vi "onHttpDelete.vi"(6 "timeout":i32=10000, 7 "output file":path, 8 "error in":errorcluster, 10 "url":string, 11 "advanced-http-client in":refnum<class "advanced-http-client.lvclass">) -> (0 "error out":errorcluster, 1 "body":string, 2 "headers":string, 3 "advanced-http-client out":refnum<class "advanced-http-client.lvclass">)   [LabVIEW 2020, in "REST Client.lvlib" / "advanced-http-client.lvclass"]
uses:
  advanced-http-client.lvclass
  advanced-http-client.lvclass/advanced-http-client.ctl
  <vilib>/NI/Advanced HTTP Client/Session.lvclass
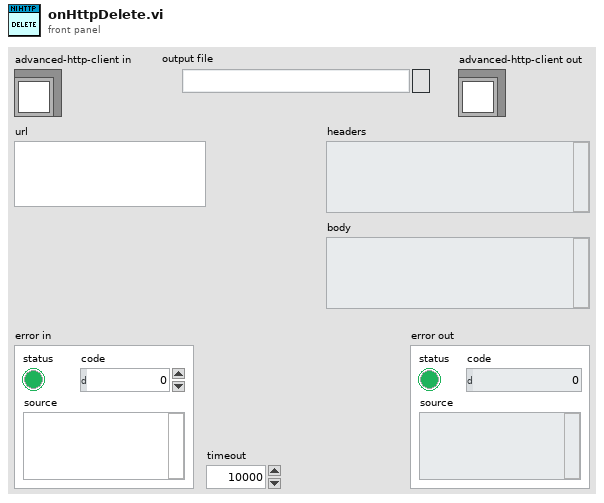
[diagram p1: front panel]
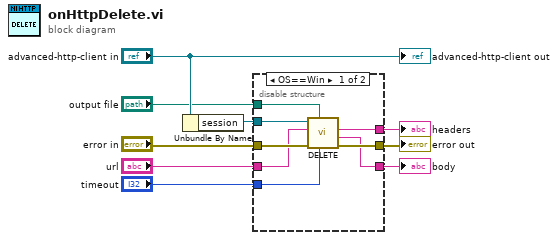
[diagram p0: block diagram]
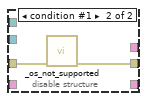
[diagram p2: hidden frame]
diagram:
  n1 = Unbundle By Name("advanced-http-client in") -> ("session"=w8:refnum<class "Session.lvclass">)
  n2 = disable-structure shown="OS==Win" {
    disable-tunnel: w8 -> [w17 _]
    disable-tunnel: "output file" -> [w16 _]
    disable-tunnel: "error in" -> [w15 w19]
    disable-tunnel: [w14 w18] -> w5
    disable-tunnel: "timeout" -> [w13 _]
    disable-tunnel: "url" -> [w12 _]
    disable-tunnel: [w11 _] -> w2
    disable-tunnel: [w10 _] -> w1
    frame condition #0 (active) {
      n3 = call <vilib>:"DELETE.vi"("timeout"=w13, "output file"=w16, "error in"=w15, "url"=w12, "session in"=w17) -> ("error out"=w14:errorcluster, "body"=w10:string, "headers"=w11:string)  [unwired: 2 in, 2 out]
    }
    frame condition #1 {
      n4 = call "_os_not_supported.vi"("error in (no error)"=w19) -> ("error out"=w18:errorcluster)  [unwired: 10 in]
    }
  }
  "error out" <- w5
  "headers" <- w2
  "body" <- w1
  "advanced-http-client out" <- "advanced-http-client in"
